vi "GEN2_Static_Read_Packs.vi"(8 "error in (no error)":errorcluster, 10 "byte expected":u32=2, 11 "VISA Refnum in":refnum<visa-resource-name>) -> (0 "error out":errorcluster, 2 "Packs":T1(array[cluster]), 3 "VISA Refnum out":refnum<visa-resource-name>)   [LabVIEW 2016, in "GEN_2.lvlib"]
uses:
  GEN_2.lvlib
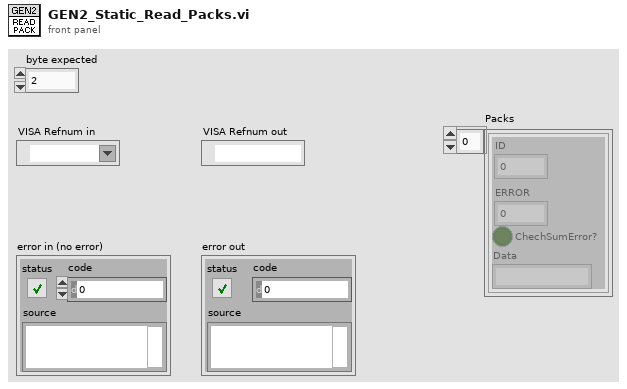
[diagram p1: front panel]
types:
  T1 = cluster{"ID":u8, "ERROR":u8, "ChechSumError?":bool, "Data":string}[]
  T2 = enum16{"big-endian, network order", "native, host order", "little-endian"}
  T3 = cluster{"ID":u8, "ERROR":u8, "ChechSumError?":bool, "Data":string}
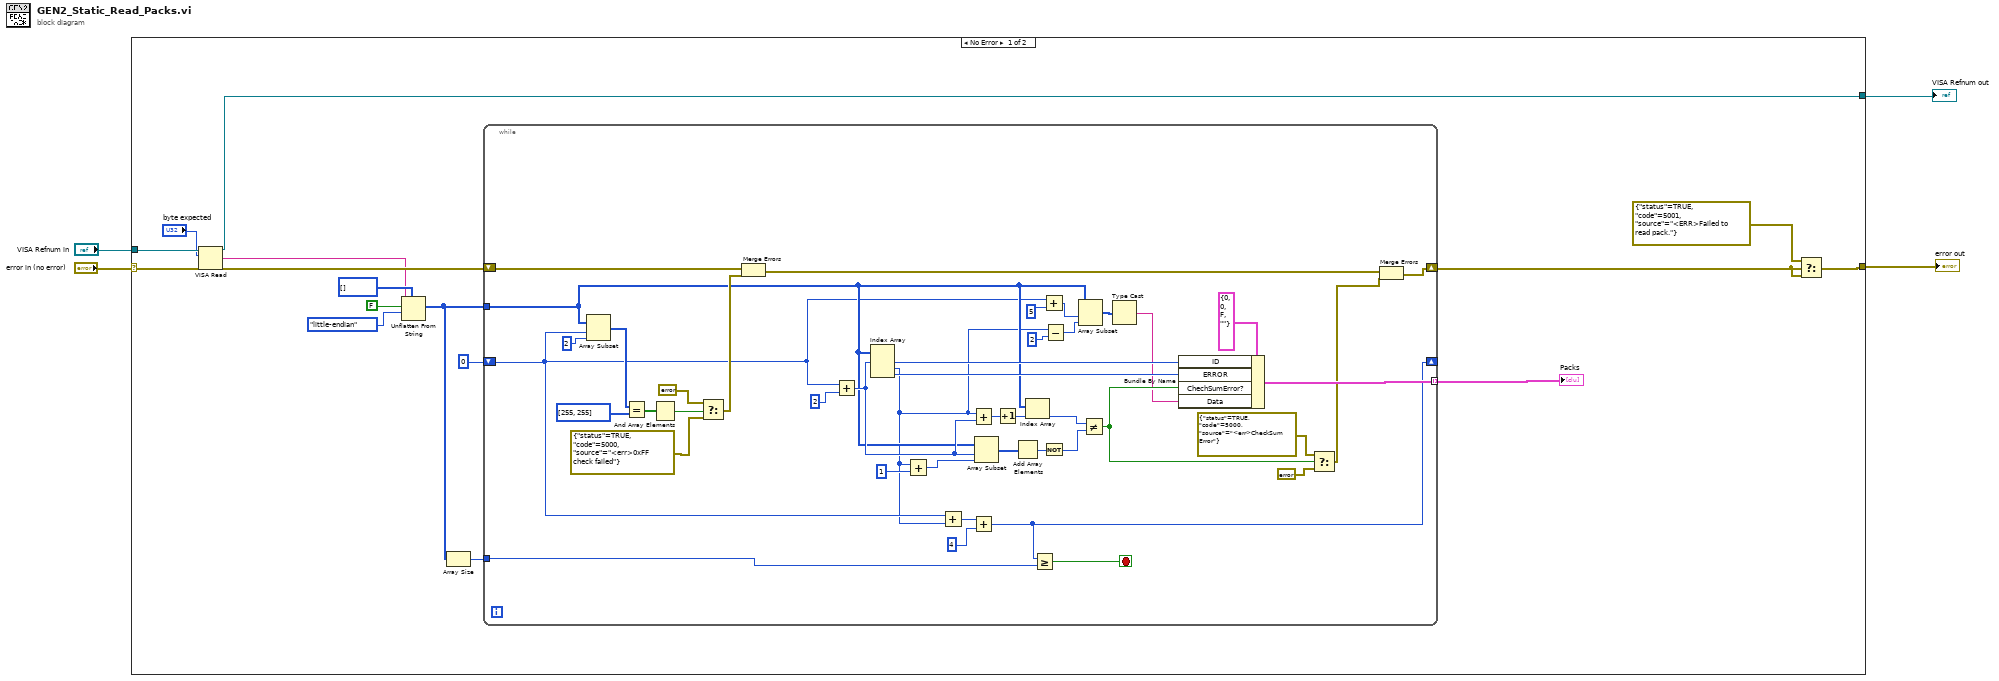
[diagram p0: block diagram]
diagram:
  n1 = case shown="No Error" "error in (no error)" {
    selector: "error in (no error)" -> [w18 w64]
    tunnel: [w9 w65] -> w4
    tunnel: [w17 w64] -> w3
    tunnel: "VISA Refnum in" -> [w20 w65]
    frame No Error {
      n2 = VISA Read(VISA resource name=w20, byte count="byte expected", error in (no error)=w18) -> (VISA resource name out=w9:refnum<visa-resource-name>, read buffer=w10:string, error out=w14:errorcluster)  [unwired: 1 out]
      n3 = Unflatten From String(type=u8[] [], binary string=w10, data includes array or string size? (T)=FALSE, byte order (0:big-endian, network order)=T2."little-endian") -> (value=w6:u8[])  [unwired: 1 in, 2 out]
      n4 = Array Size(array=w6) -> (size(s)=w5:i32)
      n5 = while {
        tunnel: [w60] -> w7 mode=indexing
        tunnel: w6 -> [w35]
        shift-right: [w57] -> w16
        shift-left: w14 -> [w51]
        shift-right: [w23] -> _
        shift-left: 0 ("index") -> [w27]
        tunnel: w5 -> [w22]
        stop <- w21 stop-if-true
        n6 = Array Subset(array=w35, index=w27, length=2 ("length (rest)")) -> (w49:u8[])
        n7 = Equal?(x=w49, y=u8[] [255, 255]) -> (x = y?=w47:bool[])
        n8 = And Array Elements(Boolean array=w47) -> (logical AND=w46:bool)
        n9 = Select(t=errorcluster {"status"=FALSE, "code"=0, "source"=""} ("No Error"), s=w46, f=errorcluster {"status"=TRUE, "code"=5000, "source"="<err>0xFF check failed"} ("FF")) -> (s? t:f=w53:errorcluster)
        n10 = Merge Errors(w51, w53) -> (w28:errorcluster)
        n11 = Add(x=w27, y=2 ("index")) -> (x+y=w40:i32)
        n12 = Index Array(array=w35, index #1=w40) -> (element #1=w61:u8, element #2=w26:u8, element #3=w44:u8)  [unwired: 2 in]
        n13 = Add(x=w26, y=u8 1) -> (x+y=w42:u8)
        n14 = Add(x=w27, y=w26) -> (x+y=w25:i32)
        n15 = Add(x=w26, y=w40) -> (x+y=w39:i32)
        n16 = Add(x=w25, y=4) -> (x+y=w23:i32)
        n17 = Array Subset(array=w35, index=w40, length=w42) -> (w41:u8[])
        n18 = Increment(x=w39) -> (x+1=w38:i32)
        n19 = Add Array Elements(numeric array=w41) -> (sum=w63:u8)
        n20 = Index Array(array=w35, index=w38) -> (element=w37:u8)
        n21 = Greater Or Equal?(x=w23, y=w22) -> (x >= y?=w21:bool)
        n22 = Add(x=w27, y=5 ("index")) -> (x+y=w33:i32)
        n23 = Not(x=w63) -> (.not. x?=w36:u8)
        n24 = Subtract(x=w26, y=u8 2) -> (x-y=w31:u8)
        n25 = Array Subset(array=w35, index=w33, length=w31) -> (w30:u8[])
        n26 = Not Equal?(x=w37, y=w36) -> (x != y?=w59:bool)
        n27 = Type Cast(x=w30) -> (*(type *) &x=w29:string)  [unwired: 1 in]
        n28 = Bundle By Name(cluster=T3 {"ID"=0, "ERROR"=0, "ChechSumError?"=FALSE, "Data"=""} ("output cluster"), "ID"=w61, "ERROR"=w44, "ChechSumError?"=w59, "Data"=w29) -> (w60:T3)
        n29 = Select(t=errorcluster {"status"=TRUE, "code"=5000, "source"="<err>CheckSum Error"} ("FF"), s=w59, f=errorcluster {"status"=FALSE, "code"=0, "source"=""}) -> (s? t:f=w58:errorcluster)
        n30 = Merge Errors(w28, w58) -> (w57:errorcluster)
      }
      "Packs" <- w7
      n31 = Select(t=errorcluster {"status"=TRUE, "code"=5001, "source"="<ERR>Failed to read pack."} ("5001"), s=w16, f=w16) -> (s? t:f=w17:errorcluster)
    }
    frame Error {
    }
  }
  "VISA Refnum out" <- w4
  "error out" <- w3
